vi "LJUD UE9RAW WriteMem.vi"(7 "Comm Settings":T1={"Open LabJack "=TRUE, "Use USB"=TRUE, "IP Address"="192.168.1.209", "PortA"=52360, "PortB"=0}, 8 "error in (no error)":errorcluster, 9 "Mem Data":u8[](array[numeric]) format="%.0x", 10 "BlockNum":u8, 11 "Handle In":i32) -> (0 "error out":errorcluster, 3 "Handle Out":i32)   [LabVIEW 2021]
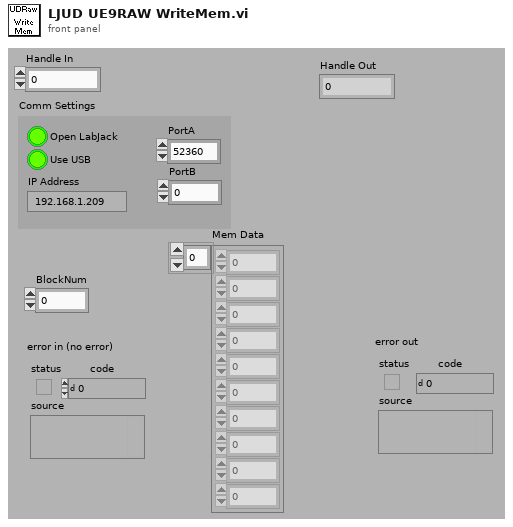
[diagram p1: front panel]
types:
  T1 = cluster{"Open LabJack ":bool, "Use USB":bool, "IP Address":string, "PortA":u16, "PortB":u16}
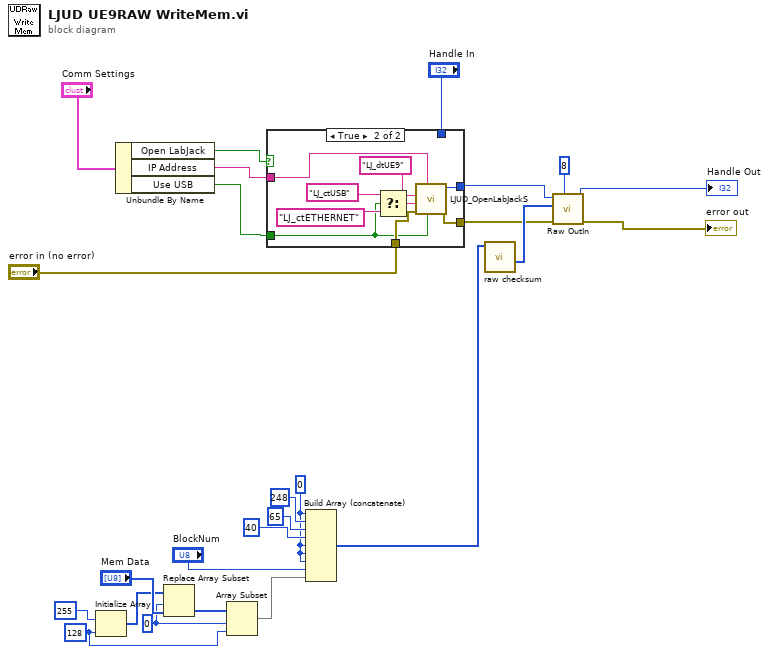
[diagram p0: block diagram]
diagram:
  w16 = 0 ("Index")
  w15 = 128 ("Dimension Size")
  w20 = u8 0 ("Input Element")
  n1 = Initialize Array(u8 255 ("Element Data"), w15) -> (w17:u8[])
  n2 = Unbundle By Name("Comm Settings") -> ("Open LabJack"=w7:bool, "IP Address"=w6:string, "Use USB"=w5:bool)
  n3 = Replace Array Subset(array=w17, new element="Mem Data", index=w16) -> (w14:u8[])
  n4 = Array Subset(array=w14, index=w16, length=w15) -> (w13:u8[])
  n5 = case shown="True" w7 {
    tunnel: w6 -> [_ w30]
    tunnel: "error in (no error)" -> [w27 w34]
    tunnel: [w27 w33] -> w3
    tunnel: [w26 w31] -> w2
    tunnel: w5 -> [_ w32]
    tunnel: "Handle In" -> [w26 _]
    frame False {
    }
    frame True {
      n6 = Select(t="LJ_ctUSB" ("ConnectionType"), s=w32, f="LJ_ctETHERNET" ("ConnectionType")) -> (s? t:f=w28:string)
      n7 = call "LJUD_OpenLabJackS.vi"("FirstFound"=w32, "Address"=w30, "error in"=w34, "ConnectionType"=w28, "DeviceType"="LJ_dtUE9") -> ("error out"=w33:errorcluster, "Handle"=w31:i32)  [unwired: 4 in, 1 out]
    }
  }
  n8 = Build Array (concatenate)(w20, u8 248 ("Input Element"), u8 65 ("Input Element"), u8 40 ("Input Element"), w20, w20, w20, "BlockNum", w13) -> (w22:u8[])
  n9 = call "raw checksum.vi"("Array"=w22) -> ("Array Output"=w12:u8[])  [unwired: 3 in, 7 out]
  n10 = call "Raw OutIn.vi"("# of bytes to read in"=8 ("# of bytes to read"), "error in"=w3, "Raw Out"=w12, "Handle In"=w2) -> ("error out"=→"error out":errorcluster, "Handle Out"=→"Handle Out":i32)  [unwired: 4 in, 2 out]
